vi "Application Globals.vi"() -> ()   [LabVIEW 2017]
panel:
  in  "RawDataQueue":refnum<queue>
  in  "DSP Queue":refnum<queue>
  in  "SpectrumQueue":refnum<queue>
  in  "Termination Notifier":refnum<notifier>
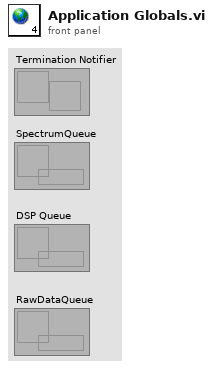
[diagram p1: front panel]
diagram:
